vi "Viavi - Multi Channel Table.vi"(7 "Channels Selected":bool[](array[boolean]), 10 "Data Input":T2) -> (0 "RL Table Output":T1(array[cluster]), 3 "Ref IL Table Output":T1(array[cluster]))   [LabVIEW 2017]
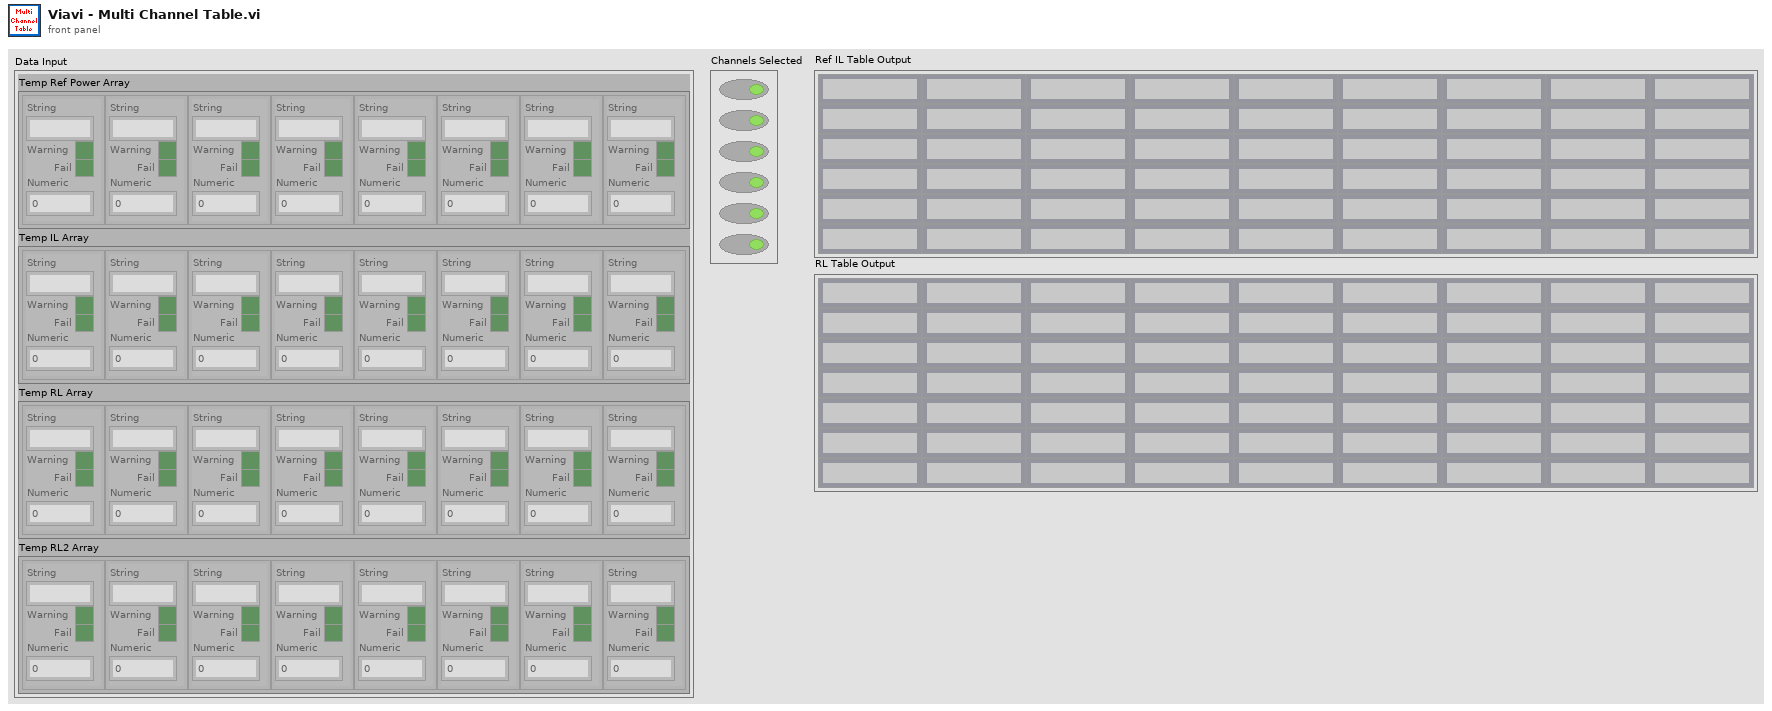
[diagram p1: front panel]
types:
  T1 = cluster{"String":string, "Warning":bool, "Fail":bool, "Numeric":dbl}[][]
  T2 = cluster{"Temp Ref Power Array":cluster{"String":string, "Warning":bool, "Fail":bool, "Numeric":dbl}[], "Temp IL Array":cluster{"String":string, "Warning":bool, "Fail":bool, "Numeric":dbl}[], "Temp RL Array":cluster{"String":string, "Warning":bool, "Fail":bool, "Numeric":dbl}[], "Temp RL2 Array":cluster{"String":string, "Warning":bool, "Fail":bool, "Numeric":dbl}[]}
  T3 = cluster{"String":string, "Warning":bool, "Fail":bool, "Numeric":dbl}[]
  T4 = cluster{"String":string, "Warning":bool, "Fail":bool, "Numeric":dbl}
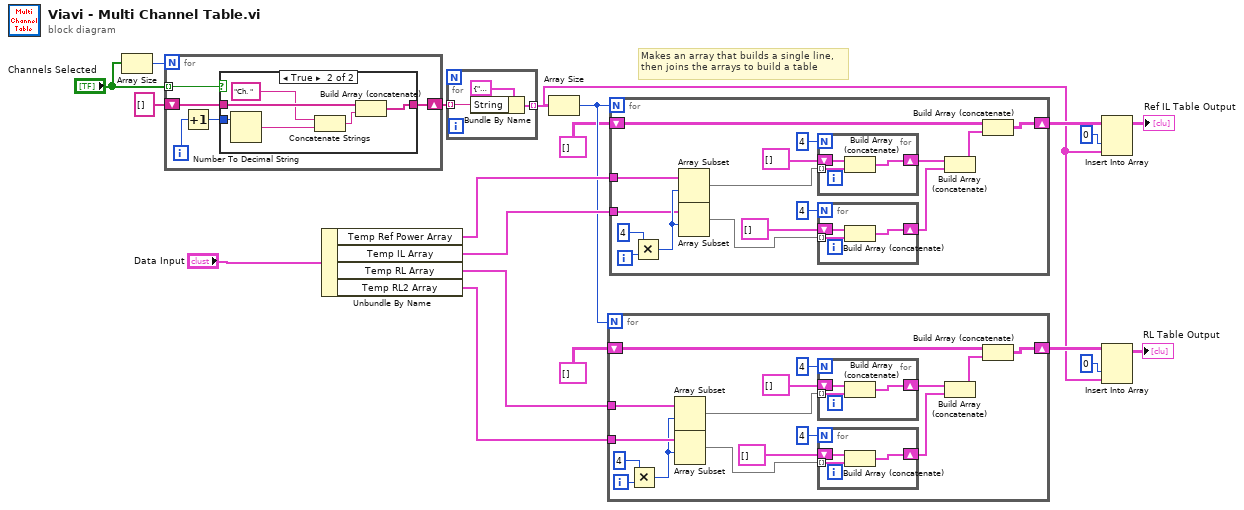
[diagram p0: block diagram]
diagram:
  # "Makes an array that builds a single line,\nthen joins the arrays to build a table"
  n1 = Array Size(array="Channels Selected") -> (size(s)=w19:i32)
  n2 = for {
    N: w19 -> [_]
    tunnel: "Channels Selected" -> [w24] mode=indexing
    shift-right: [w21] -> w2
    shift-left: string[] [] -> [w20]
    i -> [w23]
    n3 = Increment(x=w23) -> (x+1=w22:i32)
    n4 = case shown="True" w24 {
      tunnel: w22 -> [_ w29]
      tunnel: [w25 w31] -> w21
      tunnel: w20 -> [w25 w30]
      frame False {
      }
      frame True {
        n5 = Number To Decimal String(number=w29) -> (decimal integer string=w27:string)  [unwired: 1 in]
        n6 = Concatenate Strings("Ch. ", w27) -> (w26:string)
        n7 = Build Array (concatenate)(w30, w26) -> (w31:string[])
      }
    }
  }
  n8 = Unbundle By Name("Data Input") -> ("Temp Ref Power Array"=w7:T3, "Temp IL Array"=w8:T3, "Temp RL Array"=w9:T3, "Temp RL2 Array"=w10:T3)
  n9 = for {
    tunnel: w2 -> [w33] mode=indexing
    tunnel: [w32] -> w1 mode=indexing
    n10 = Bundle By Name(cluster=T4 {"String"="", "Warning"=FALSE, "Fail"=FALSE, "Numeric"=0.0} ("Single Cell Cluster"), "String"=w33) -> (w32:T4)
  }
  n11 = Array Size(array=w1) -> (size(s)=w6:i32)
  n12 = for {
    N: w6 -> [_]
    tunnel: w9 -> [w43]
    shift-right: [w45] -> w15
    shift-left: T1 [] -> [w44]
    tunnel: w10 -> [w42]
    i -> [w41]
    n13 = Multiply(x=4, y=w41) -> (x*y=w39:i32)
    n14 = Array Subset(array=w43, index=w39) -> (w38:T3)  [unwired: 1 in]
    n15 = Array Subset(array=w42, index=w39) -> (w37:T3)  [unwired: 1 in]
    n16 = for {
      N: 4 -> [_]
      tunnel: w38 -> [w56] mode=indexing
      shift-right: [w55] -> w47
      shift-left: T3 [] -> [w54]
      n17 = Build Array (concatenate)(w54, w56) -> (w55:T3)
    }
    n18 = for {
      N: 4 -> [_]
      tunnel: w37 -> [w53] mode=indexing
      shift-right: [w52] -> w48
      shift-left: T3 [] -> [w51]
      n19 = Build Array (concatenate)(w51, w53) -> (w52:T3)
    }
    n20 = Build Array (concatenate)(w47, w48) -> (w46:T3)
    n21 = Build Array (concatenate)(w44, w46) -> (w45:T1)
  }
  n22 = for {
    N: w6 -> [_]
    tunnel: w7 -> [w64]
    shift-right: [w57] -> w11
    shift-left: T1 [] -> [w67]
    tunnel: w8 -> [w63]
    i -> [w62]
    n23 = Multiply(x=4, y=w62) -> (x*y=w65:i32)
    n24 = Array Subset(array=w64, index=w65) -> (w60:T3)  [unwired: 1 in]
    n25 = Array Subset(array=w63, index=w65) -> (w61:T3)  [unwired: 1 in]
    n26 = for {
      N: 4 -> [_]
      tunnel: w60 -> [w78] mode=indexing
      shift-right: [w77] -> w69
      shift-left: T3 [] -> [w76]
      n27 = Build Array (concatenate)(w76, w78) -> (w77:T3)
    }
    n28 = for {
      N: 4 -> [_]
      tunnel: w61 -> [w75] mode=indexing
      shift-right: [w74] -> w70
      shift-left: T3 [] -> [w73]
      n29 = Build Array (concatenate)(w73, w75) -> (w74:T3)
    }
    n30 = Build Array (concatenate)(w69, w70) -> (w68:T3)
    n31 = Build Array (concatenate)(w67, w68) -> (w57:T1)
  }
  n32 = Insert Into Array(array=w11, index (col)=0 ("index (row)"), new element=w1) -> (→"Ref IL Table Output":T1)  [unwired: 1 in]
  n33 = Insert Into Array(array=w15, index (col)=0 ("index (row)"), new element=w1) -> (→"RL Table Output":T1)  [unwired: 1 in]
